vi "Format Multi Waveform Graph.vi"(0 "sample rate (Hz)":dbl=250000000.0 format="%#_6p", 1 "array of chans":u32[](array[numeric]), 2 "waveform graph":refnum<vi>, 5 "data in":dbl[][](graph), 7 "relativeX (samples)":dbl[](array[numeric]), 9 "start record number":u64, 11 "error in":errorcluster) -> (4 "waveform out":T1(graph), 15 "error out":errorcluster)   [LabVIEW 2021]
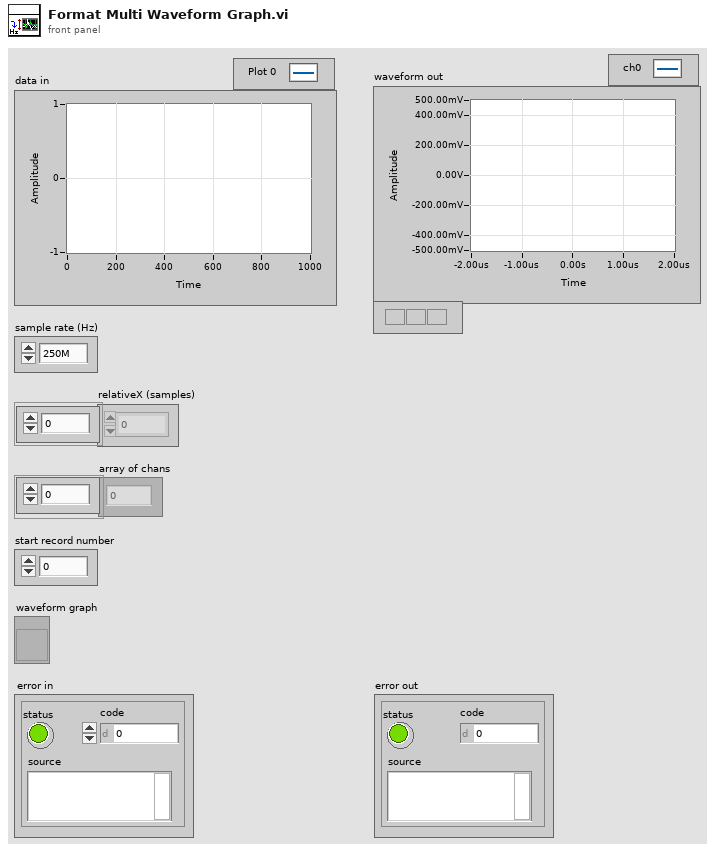
[diagram p1: front panel]
types:
  T1 = cluster{"relativeX":dbl, "sample rate":dbl, "data in":dbl[]}[]
  T2 = cluster{"relativeX":dbl, "sample rate":dbl, "data in":dbl[]}
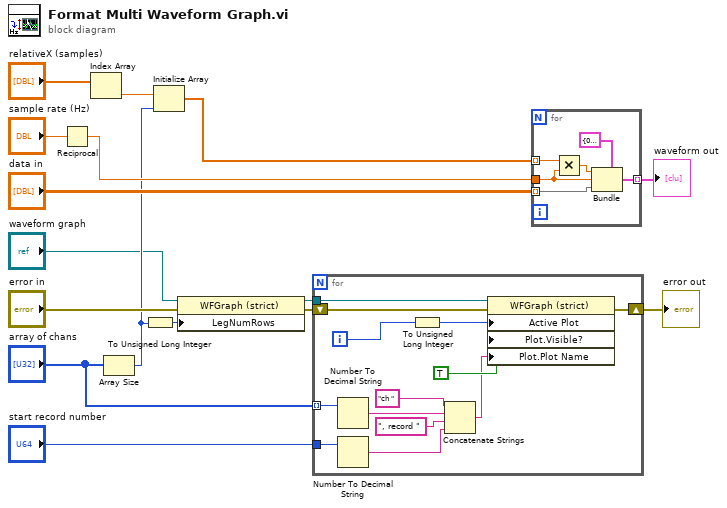
[diagram p0: block diagram]
diagram:
  n1 = Reciprocal(x="sample rate (Hz)") -> (1/x=w14:dbl)
  n2 = Index Array(array="relativeX (samples)") -> (element=w4:dbl)  [unwired: 1 in]
  n3 = Array Size(array="array of chans") -> (size(s)=w5:i32)
  n4 = To Unsigned Long Integer(number=w5) -> (unsigned 32bit integer=w7:u32)
  n5 = Initialize Array(w4, w5) -> (w3:dbl[])
  n6 = property on="Property Node" class="WFGraph (strict)"(reference="waveform graph", error in="error in", "LegNumRows"=w7) -> (reference out=w9:refnum<vi>, error out=w10:errorcluster)
  n7 = for {
    tunnel: w9 -> [w23]
    shift-right: [w19] -> w11
    shift-left: w10 -> [w20]
    tunnel: "start record number" -> [w18]
    tunnel: "array of chans" -> [w17] mode=indexing
    i -> [w22]
    n8 = Number To Decimal String(number=w17) -> (decimal integer string=w25:string)  [unwired: 1 in]
    n9 = Number To Decimal String(number=w18) -> (decimal integer string=w28:string)  [unwired: 1 in]
    n10 = To Unsigned Long Integer(number=w22) -> (unsigned 32bit integer=w21:u32)
    n11 = Concatenate Strings("ch " ("Plot.Plot Name"), w25, ", record " ("string"), w28) -> (w24:string)
    n12 = property on="Property Node" class="WFGraph (strict)"(reference=w23, error in=w20, "Active Plot"=w21, "Plot.Visible?"=TRUE ("Plot.Visible"), "Plot.Plot Name"=w24) -> (error out=w19:errorcluster)  [unwired: 1 out]
  }
  "error out" <- w11
  n13 = for {
    tunnel: "data in" -> [w35] mode=indexing
    tunnel: w14 -> [w32]
    tunnel: [w34] -> w1 mode=indexing
    tunnel: w3 -> [w31] mode=indexing
    n14 = Multiply(x=w31, y=w32) -> (x*y=w33:dbl)
    n15 = Bundle(cluster=T2 {"relativeX"=0.0, "sample rate"=0.0, "data in"=[]}, "relativeX"=w33, "sample rate"=w32, "data in"=w35) -> (w34:T2)
  }
  "waveform out" <- w1
